vi "nivsfpga_Create Project.vi"(8 "error in (no error)":errorcluster, 10 "project filename":path, 11 "Custom FPGA Name":string) -> (0 "error out":errorcluster)   [LabVIEW 2010]
uses:
  <userlib>/_NI VeriStand FPGA Support/NI VeriStand FPGA Template Tool/ProjectWizard/subVIs/nivsfpga_Reference Global.vi
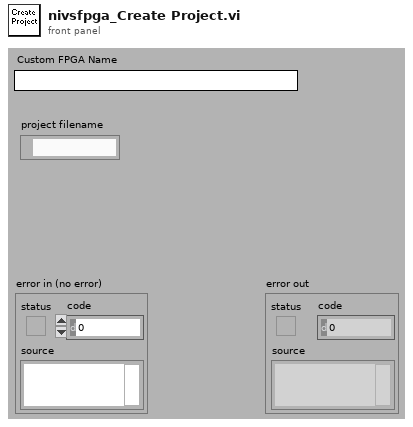
[diagram p1: front panel]
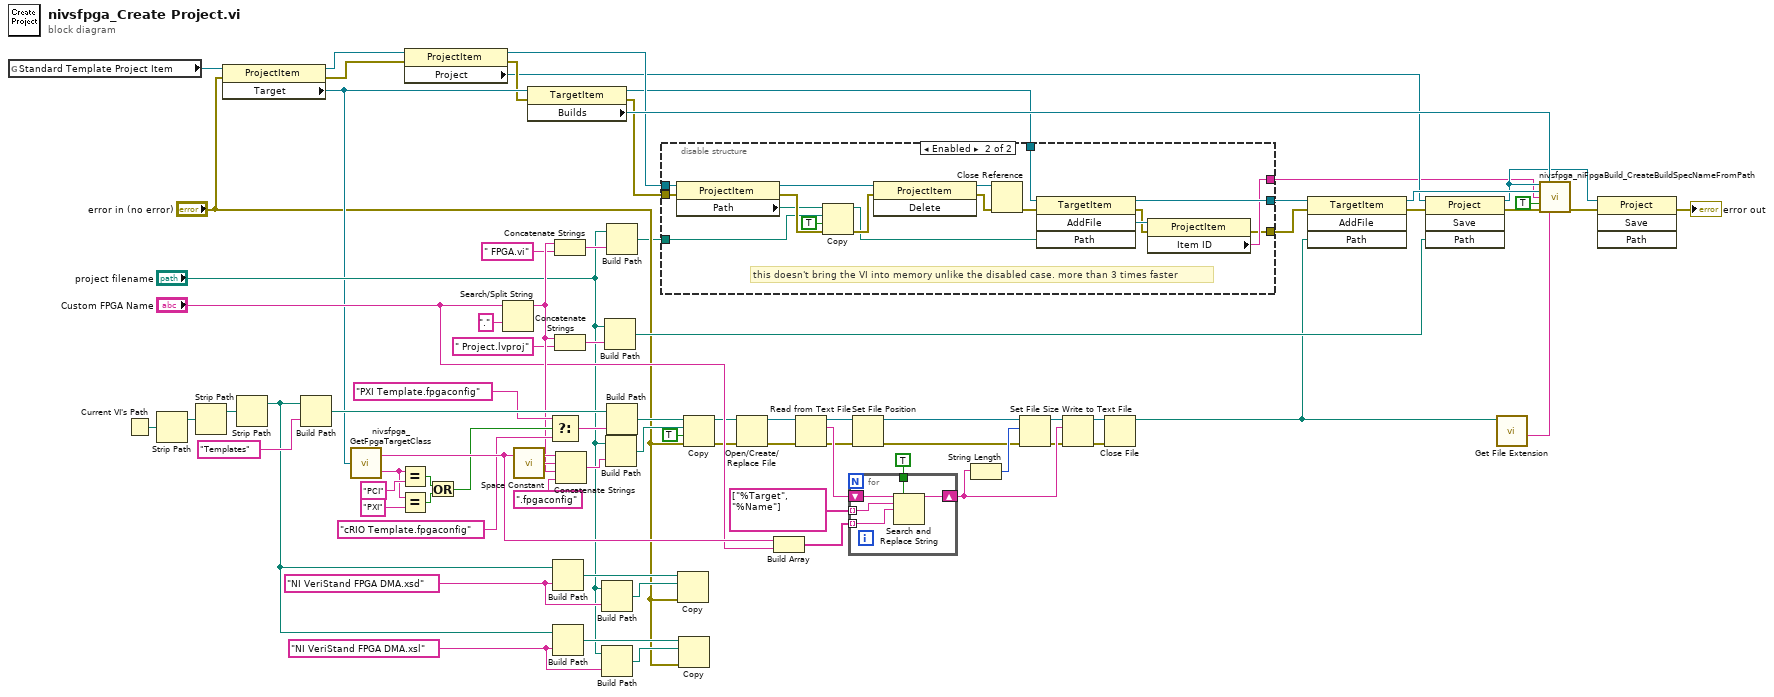
[diagram p0: block diagram]
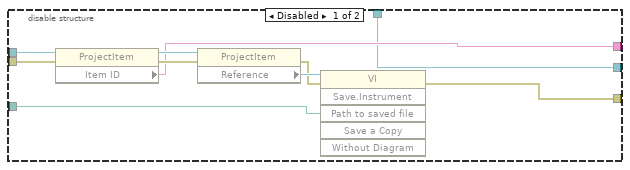
[diagram p2: hidden frame]
diagram:
  w50 = "NI VeriStand FPGA DMA.xsl" ("name or relative path")
  w46 = "NI VeriStand FPGA DMA.xsd" ("name or relative path")
  n1 = global read "nivsfpga_Reference Global.vi" "Standard Template Project Item"() -> (w21:refnum<vi>)
  n2 = Current VI's Path() -> (path=w31:path)
  n3 = Strip Path(path=w31) -> (stripped path=w30:path)  [unwired: 1 out]
  n4 = Strip Path(path=w30) -> (stripped path=w40:path)  [unwired: 1 out]
  n5 = property class="ProjectItem"(reference=w21, error in="error in (no error)") -> (reference out=w6:refnum<vi>, error out=w7:errorcluster, "Target"=w25:refnum<vi>)
  n6 = Strip Path(path=w40) -> (stripped path=w27:path)  [unwired: 1 out]
  n7 = Build Path(base path=w27, name or relative path="Templates") -> (appended path=w62:path)
  n8 = call <userlib>:"nivsfpga_GetFpgaTargetClass.vi"("FPGA target"=w25) -> ("Target"=w75:string, "Platform"=w55:string)
  n9 = Equal?(x=w55, y="PCI") -> (x = y?=w58:bool)
  n10 = Equal?(x=w55, y="PXI") -> (x = y?=w59:bool)
  n11 = property class="ProjectItem"(reference=w6, error in=w7) -> (reference out=w10:refnum<vi>, error out=w20:errorcluster, "Project"=w8:refnum<vi>)
  n12 = Or(x=w58, y=w59) -> (x .or. y?=w60:bool)
  n13 = Search/Split String(string="Custom FPGA Name", search string/char (-)=".") -> (substring before match=w51:string)  [unwired: 1 in, 2 out]
  n14 = call <vilib>:"Space Constant.vi"() -> ("String"=w52:string)
  n15 = property class="TargetItem"(reference=w25, error in=w20) -> (reference out=w5:refnum<vi>, error out=w11:errorcluster, "Builds"=w24:refnum<vi>)
  n16 = Select(t="PXI Template.fpgaconfig" ("name or relative path"), s=w60, f="cRIO Template.fpgaconfig" ("name or relative path")) -> (s? t:f=w53:string)
  n17 = Build Path(base path=w27, name or relative path=w46) -> (appended path=w45:path)
  n18 = Build Path(base path=w27, name or relative path=w50) -> (appended path=w49:path)
  n19 = Concatenate Strings(w51, " FPGA.vi" ("string")) -> (w38:string)
  n20 = Concatenate Strings(w51, " Project.lvproj" ("string")) -> (w34:string)
  n21 = Concatenate Strings(w75, w52, w51, ".fpgaconfig" ("string")) -> (w43:string)
  n22 = Build Path(base path="project filename", name or relative path=w46) -> (appended path=w48:path)
  n23 = Build Path(base path="project filename", name or relative path=w50) -> (appended path=w47:path)
  n24 = Build Path(base path="project filename", name or relative path=w34) -> (appended path=w37:path)
  n25 = Build Path(base path="project filename", name or relative path=w43) -> (appended path=w42:path)
  n26 = Build Path(base path="project filename", name or relative path=w38) -> (appended path=w9:path)
  n27 = Build Path(base path=w62, name or relative path=w53) -> (appended path=w41:path)
  n28 = disable-structure shown="Enabled" {
    disable-tunnel: [w87 w91] -> w16
    disable-tunnel: w11 -> [w84 w103]
    disable-tunnel: w10 -> [w85 w102]
    disable-tunnel: w9 -> [w86 w101]
    disable-tunnel: w5 -> [w80 w96]
    disable-tunnel: [w80 w95] -> w4
    disable-tunnel: [w81 w92] -> w3
    frame Disabled {
      n29 = property class="ProjectItem"(reference=w85, error in=w84) -> (reference out=w82:refnum<vi>, error out=w83:errorcluster, "Item ID"=w81:string)
      n30 = property class="ProjectItem"(reference=w82, error in=w83) -> (error out=w88:errorcluster, "Reference"=w89:refnum<vi>)  [unwired: 1 out]
      n31 = invoke class="VI" method="Save.Instrument"(reference=w89, error in=w88, "Path to saved file"=w86) -> (error out=w87:errorcluster)  [unwired: 3 in, 5 out]
    }
    frame Enabled {
      # "this doesn't bring the VI into memory unlike the disabled case. more than 3 times faster"
      n32 = property class="ProjectItem"(reference=w102, error in=w103) -> (reference out=w106:refnum<vi>, error out=w105:errorcluster, "Path"=w90:path)
      n33 = Copy(8:w105, 9:TRUE ("overwrite (F)"), 10:w101, 11:w90) -> (0:w107:errorcluster, 3:w97:path)  [unwired: 2 out]
      n34 = invoke class="ProjectItem" method="Delete"(reference=w106, error in=w107) -> (reference out=w100:refnum<vi>, error out=w99:errorcluster)  [unwired: 1 in, 1 out]
      n35 = Close Reference(reference=w100, error in (no error)=w99) -> (error out=w98:errorcluster)
      n36 = invoke class="TargetItem" method="AddFile"(reference=w96, error in=w98, "Path"=w97) -> (reference out=w95:refnum<vi>, error out=w93:errorcluster, "AddFile"=w94:refnum<vi>)  [unwired: 1 in, 1 out]
      n37 = property class="ProjectItem"(reference=w94, error in=w93) -> (error out=w91:errorcluster, "Item ID"=w92:string)  [unwired: 1 out]
    }
  }
  n38 = Copy(8:"error in (no error)", 10:w48, 11:w45) -> ()  [unwired: 1 in, 4 out]
  n39 = Copy(8:"error in (no error)", 10:w47, 11:w49) -> ()  [unwired: 1 in, 4 out]
  n40 = Copy(8:"error in (no error)", 9:TRUE ("overwrite (F)"), 10:w42, 11:w41) -> (0:w22:errorcluster, 3:w28:path)  [unwired: 2 out]
  n41 = Open/Create/Replace File(file path (use dialog)=w28, error in=w22) -> (refnum out=w72:refnum<file>, error out=w29:errorcluster)  [unwired: 5 out]
  n42 = Build Array(w75, "Custom FPGA Name") -> (w76:string[])
  n43 = Read from Text File(file (use dialog)=w72, error in=w29) -> (refnum out=w71:refnum<file>, text=w74:string, error out=w70:errorcluster)  [unwired: 3 out]
  n44 = for {
    tunnel: string[] ["%Target", "%Name"] -> [w111] mode=indexing
    shift-right: [w109] -> w79
    shift-left: w74 -> [w112]
    tunnel: w76 -> [w110] mode=indexing
    tunnel: TRUE ("replace all? (F)") -> [w108]
    n45 = Search and Replace String(replace all?=w108, input string=w112, search string=w111, replace string=w110) -> (result string=w109:string)  [unwired: 1 in, 6 out]
  }
  n46 = Set File Position(refnum=w71, error in=w70) -> (refnum out=w69:refnum<file>, error out=w68:errorcluster)  [unwired: 2 out]
  n47 = String Length(string=w79) -> (length=w78:i32)
  n48 = Set File Size(4:w68, 6:w78, 7:w69) -> (0:w66:errorcluster, 3:w67:refnum<file>)
  n49 = Write to Text File(file (use dialog)=w67, text=w79, error in=w66) -> (refnum out=w64:refnum<file>, error out=w65:errorcluster)  [unwired: 2 out]
  n50 = Close File(refnum=w64, error in=w65) -> (path=w2:path)  [unwired: 1 out]
  n51 = invoke class="TargetItem" method="AddFile"(reference=w4, error in=w16, "Path"=w2) -> (reference out=w18:refnum<vi>, error out=w15:errorcluster)  [unwired: 1 in, 2 out]
  n52 = invoke class="Project" method="Save"(reference=w8, error in=w15, "Path"=w37) -> (reference out=w17:refnum<vi>, error out=w14:errorcluster)  [unwired: 1 in, 2 out]
  n53 = call <vilib>:"Get File Extension.vi"("file"=w2) -> ("filename without extension"=w1:string)  [unwired: 7 in, 3 out]
  n54 = call <userlib>:"nivsfpga_niFpgaBuild_CreateBuildSpecNameFromPath.vi"("Project"=w17, "Build Spec"=w24, "FPGA Target"=w18, "vi item ID"=w3, "make default"=TRUE, "error in (no error)"=w14, "bitfile name"=w1) -> ("error out"=w13:errorcluster)  [unwired: 7 in, 1 out]
  n55 = invoke class="Project" method="Save"(reference=w17, error in=w13) -> (error out=→"error out":errorcluster)  [unwired: 2 in, 3 out]
